vi "DAQmxAcqMessageLoop.vi"(8 "Error In":errorcluster, 11 "CommunicationRefs":T1) -> (0 "Error Out":errorcluster)   [LabVIEW 2015]
uses:
  TypeDefs/CommunicationRefs.ctl
  TypeDefs/MessageCluster.ctl
  TypeDefs/DAQmxAcqSettings.ctl
  <vilib>/DAQmx/read.llb/DAQmx Read (Analog 1D DBL 1Chan NSamp).vi
  <vilib>/Analysis/baseanly.llb/Mean (DBL).vi
  <vilib>/DAQmx/create/channels.llb/DAQmx Create Channel (AI-Temperature-Thermocouple).vi
  <vilib>/DAQmx/configure/timing.llb/DAQmx Timing (Sample Clock).vi
  <vilib>/DAQmx/miscellaneous.llb/DAQmx Fill In Error Info.vi
  <vilib>/Analysis/NI_AALBase.lvlib
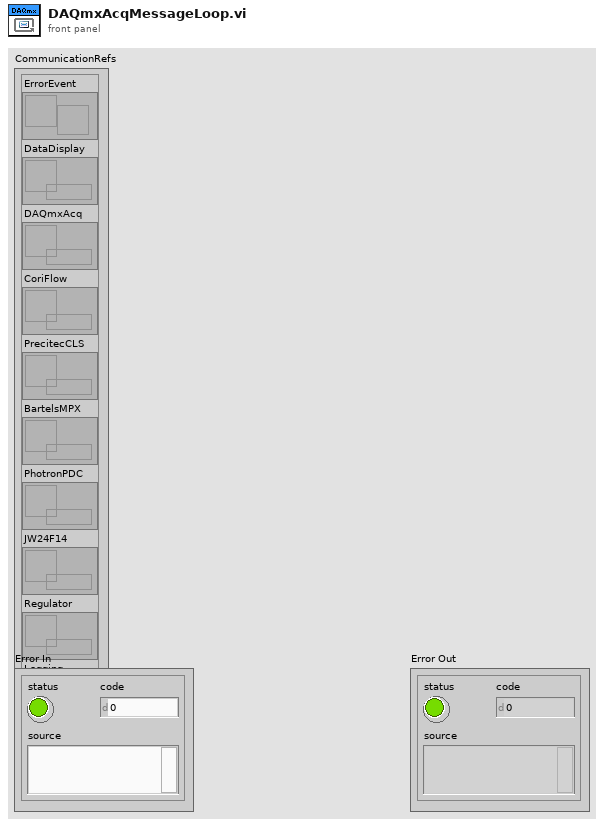
[diagram p1: front panel]
types:
  T1 = typedef "CommunicationRefs.ctl" = cluster{"ErrorEvent":refnum<user-event>, "DataDisplay":refnum<queue>, "DAQmxAcq":refnum<queue>, "CoriFlow":refnum<queue>, "PrecitecCLS":refnum<queue>, "BartelsMPX":refnum<queue>, "PhotronPDC":refnum<queue>, "JW24F14":refnum<queue>, "Regulator":refnum<queue>, "Logging":refnum<queue>}
  T2 = typedef "DAQmxAcqSettings.ctl" = cluster{"DAQmx Channel":tag, "Min Temp":dbl, "Max Temp":dbl, "Thermocouple Type":i32, "Simulate":bool, "Temp Unit":i32}
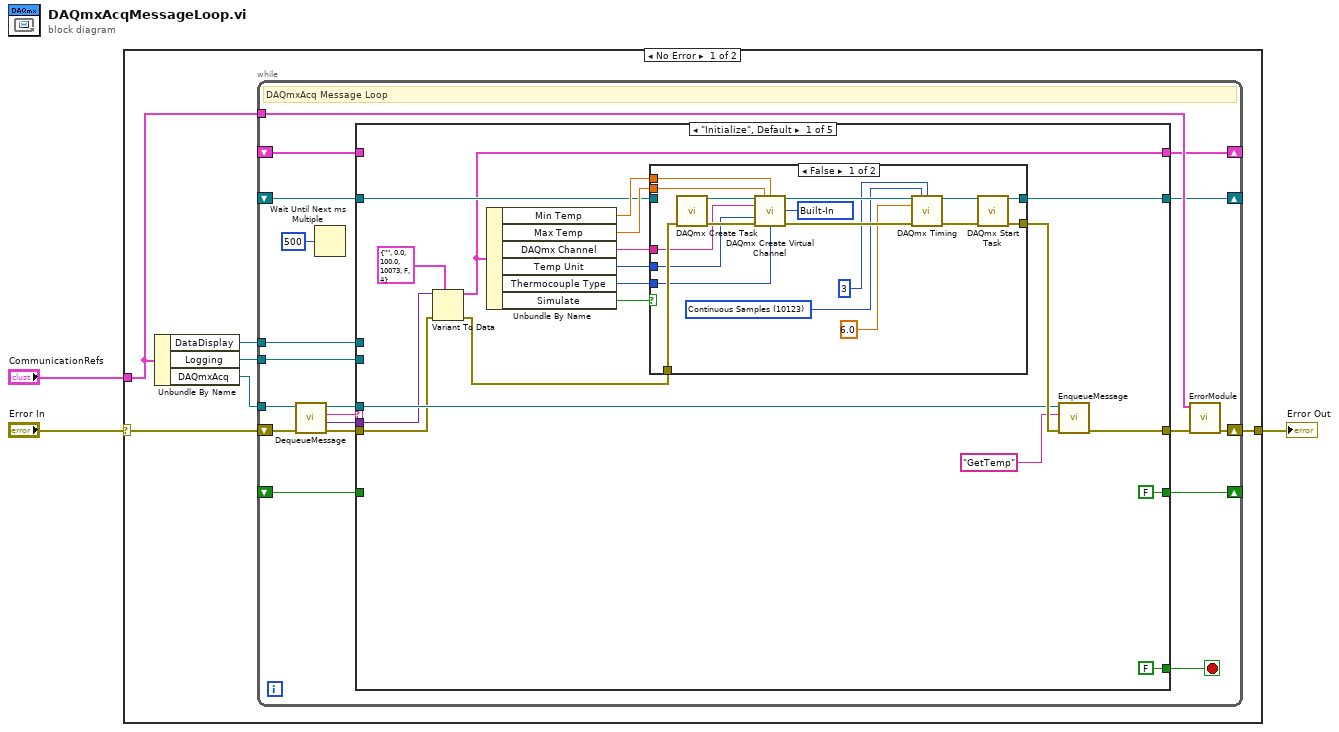
[diagram p0: block diagram]
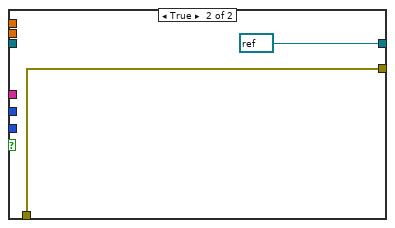
[diagram p2: hidden frame]
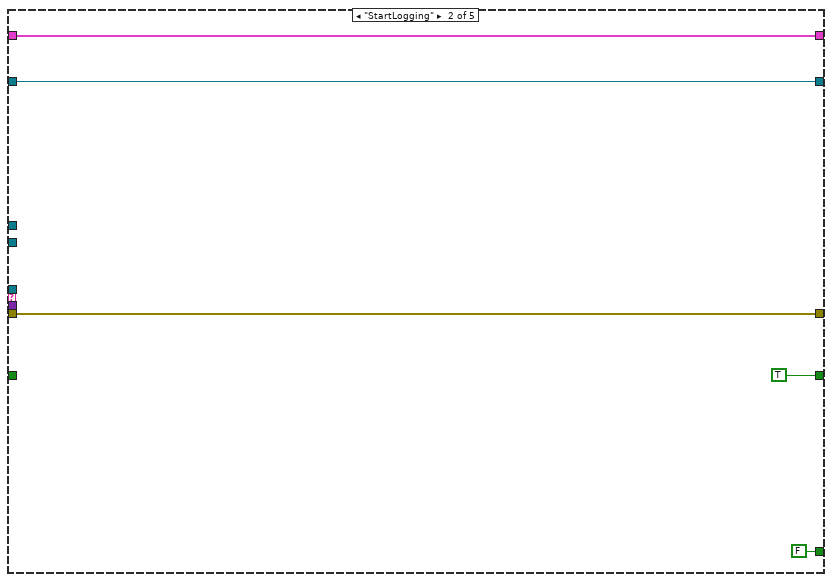
[diagram p3: hidden frame]
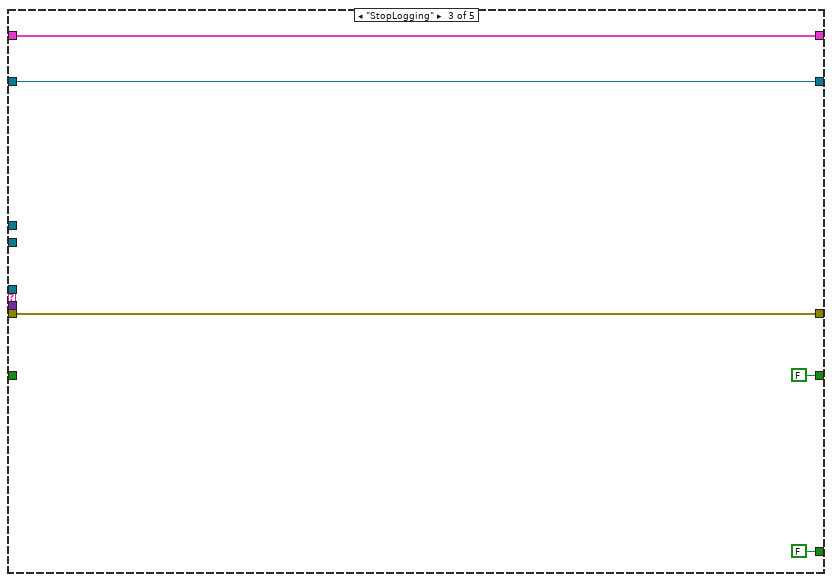
[diagram p4: hidden frame]
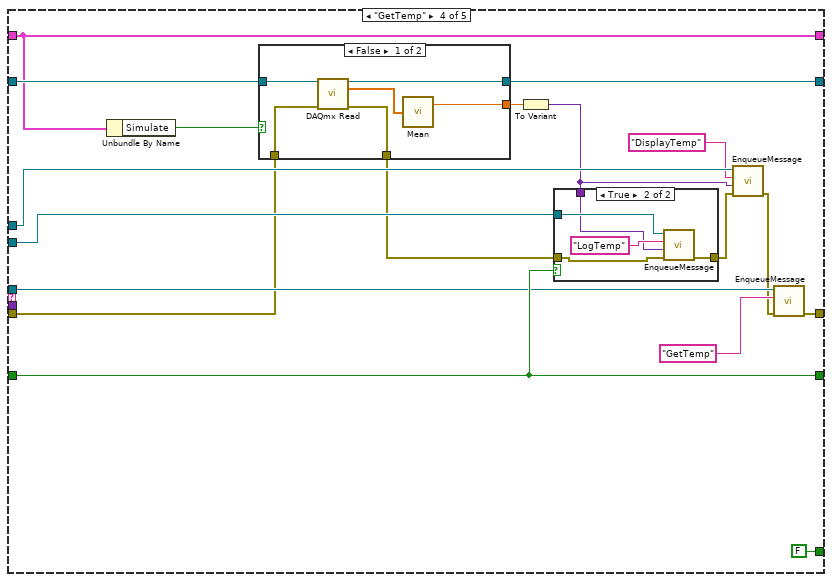
[diagram p5: hidden frame]
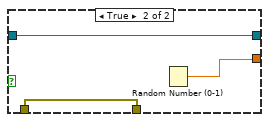
[diagram p6: hidden frame]
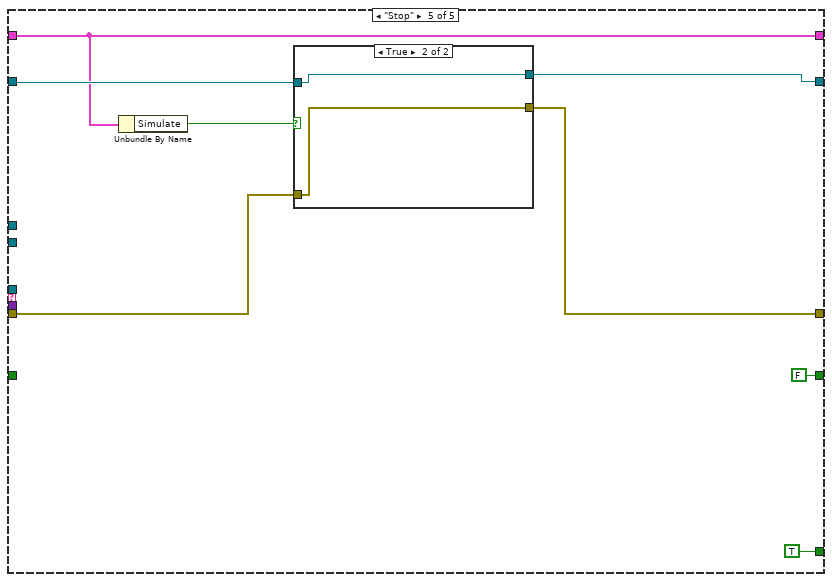
[diagram p8: hidden frame]
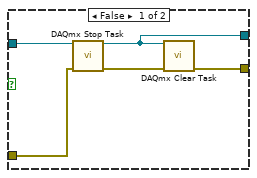
[diagram p9: hidden frame]
diagram:
  n1 = case shown="No Error" "Error In" {
    selector: "Error In" -> [w8 w126]
    tunnel: [w7 w126] -> w2
    tunnel: "CommunicationRefs" -> [w6 _]
    frame No Error {
      n2 = Unbundle By Name(w6) -> ("DataDisplay"=w5:refnum<queue>, "Logging"=w4:refnum<queue>, "DAQmxAcq"=w9:refnum<queue>)
      n3 = while {
        tunnel: w9 -> [w28]
        tunnel: w6 -> [w20]
        shift-right: [w22] -> w7
        shift-left: w8 -> [w27]
        tunnel: w5 -> [w18]
        tunnel: w4 -> [w17]
        shift-right: [w16] -> _
        shift-left: _ -> [w15]
        shift-right: [w14] -> _
        shift-left: _ -> [w13]
        shift-right: [w12] -> _
        shift-left: _ -> [w11]
        stop <- w19 stop-if-true
        # "DAQmxAcq Message Loop"
        n4 = call "DequeueMessage.vi"("error in (no error)"=w27, "MessageQueue"=w28) -> ("error out"=w23:errorcluster, "MessageData"=w24:variant, "Message"=w25:string, "dupMessageQueue"=w26:refnum<queue>)  [unwired: 6 in]
        n5 = Wait Until Next ms Multiple(millisecond multiple=u32 500) -> ()  [unwired: 1 out]
        n6 = case shown="\"Initialize\", Default" w25 {
          tunnel: w26 -> [w43 _ _ w87 _]
          tunnel: w24 -> [w40 _ _ _ _]
          tunnel: w23 -> [w41 w71 w77 w81 w112]
          tunnel: [w44 w71 w77 w88 w111] -> w21
          tunnel: [FALSE FALSE FALSE FALSE TRUE] -> w19
          tunnel: w18 -> [_ _ _ w94 _]
          tunnel: w17 -> [_ _ _ w95 _]
          tunnel: [FALSE TRUE FALSE w91 FALSE] -> w16
          tunnel: w15 -> [_ _ _ w91 _]
          tunnel: [w39 w69 w74 w82 w115] -> w14
          tunnel: w13 -> [w34 w69 w74 w90 w116]
          tunnel: [w32 w68 w73 w83 w114] -> w12
          tunnel: w11 -> [_ w68 w73 w83 w114]
          frame "Initialize", Default {
            n7 = Variant To Data(error in=w41, type=T2 {"DAQmx Channel"="", "Min Temp"=0.0, "Max Temp"=100.0, "Thermocouple Type"=10073, "Simulate"=FALSE, "Temp Unit"=4} ("DAQmxAcq Settings"), Variant=w40) -> (data=w32:T2, error out=w38:errorcluster)
            n8 = Unbundle By Name(w32) -> ("Min Temp"=w37:dbl, "Max Temp"=w36:dbl, "DAQmx Channel"=w35:tag, "Temp Unit"=w30:i32, "Thermocouple Type"=w31:i32, "Simulate"=w29:bool)
            n9 = case shown="False" w29 {
              tunnel: [w59 w67] -> w45
              tunnel: [w58 refnum<k21> refnum ("task out")] -> w39
              tunnel: w38 -> [w57 w67]
              tunnel: w37 -> [w56 _]
              tunnel: w36 -> [w55 _]
              tunnel: w35 -> [w54 _]
              tunnel: w34 -> [_ _]
              tunnel: w31 -> [w49 _]
              tunnel: w30 -> [w48 _]
              frame False {
                w51 = 10123 items=["Finite Samples"=10178, "Continuous Samples"=10123, "Hardware Timed Single Point"=12522] ("sample mode")
                w53 = 10200 items=["Built-In"=10200, "Constant Value"=10116, "Channel"=10113] ("cjc source")
                n10 = call <vilib>:"DAQmx Create Task.vi"("error in"=w57) -> ("task out"=w65:refnum<k21>, "error out"=w62:errorcluster)  [unwired: 13 in]
                n11 = call-poly <vilib>:"DAQmx Create Virtual Channel.vi"("task in"=w65, "maximum value"=w55, "minimum value"=w56, "physical channels"=w54, "cjc source"=w53, "units"=w48, "error in"=w62, "thermocouple type"=w49) -> ("task out"=w64:refnum<k21>, "error out"=w61:errorcluster)  [unwired: 6 in]
                n12 = call-poly <vilib>:"DAQmx Timing.vi"("task/channels in"=w64, "sample mode"=w51, "samples per channel"=3, "rate"=6.0, "error in"=w61) -> ("task out"=w63:refnum<k21>, "error out"=w60:errorcluster)  [unwired: 9 in]
                n13 = call <vilib>:"DAQmx Start Task.vi"("task/channels in"=w63, "error in"=w60) -> ("task out"=w58:refnum<k21>, "error out"=w59:errorcluster)  [unwired: 12 in]
              }
              frame True {
              }
            }
            n14 = call "EnqueueMessage.vi"("error in (no error)"=w45, "Message"="GetTemp", "MessageQueue"=w43) -> ("error out"=w44:errorcluster)  [unwired: 7 in, 1 out]
          }
          frame "StartLogging" {
          }
          frame "StopLogging" {
          }
          frame "GetTemp" {
            n15 = Unbundle By Name(w83) -> ("Simulate"=w89:bool)
            n16 = case shown="False" w89 {
              tunnel: w90 -> [w100 w103]
              tunnel: [w99 w104] -> w85
              tunnel: [w98 w103] -> w82
              tunnel: w81 -> [w97 w102]
              tunnel: [w96 w102] -> w80
              frame False {
                n17 = call-poly <vilib>:"DAQmx Read.vi"("task/channels in"=w100, "error in"=w97) -> ("task out"=w98:refnum<k21>, "data"=w101:dbl[], "error out"=w96:errorcluster)  [unwired: 11 in]
                n18 = call-poly <vilib>:"Mean.vi"("X"=w101) -> ("mean"=w99:dbl)  [unwired: 1 out]
              }
              frame True {
                n19 = Random Number (0-1)() -> (number: 0 to 1=w104:dbl)
              }
            }
            n20 = To Variant(anything=w85) -> (Variant=w84:variant)
            n21 = case shown="True" w91 {
              tunnel: w95 -> [_ w110]
              tunnel: w80 -> [w105 w107]
              tunnel: [w105 w106] -> w79
              tunnel: w84 -> [_ w108]
              frame False {
              }
              frame True {
                n22 = call "EnqueueMessage.vi"("error in (no error)"=w107, "MessageData"=w108, "Message"="LogTemp", "MessageQueue"=w110) -> ("error out"=w106:errorcluster)  [unwired: 6 in, 1 out]
              }
            }
            n23 = call "EnqueueMessage.vi"("error in (no error)"=w79, "MessageData"=w84, "Message"="DisplayTemp", "MessageQueue"=w94) -> ("error out"=w78:errorcluster)  [unwired: 6 in, 1 out]
            n24 = call "EnqueueMessage.vi"("error in (no error)"=w78, "Message"="GetTemp", "MessageQueue"=w87) -> ("error out"=w88:errorcluster)  [unwired: 7 in, 1 out]
          }
          frame "Stop" {
            n25 = Unbundle By Name(w114) -> ("Simulate"=w113:bool)
            n26 = case shown="True" w113 {
              tunnel: w116 -> [w123 w124]
              tunnel: [w122 w124] -> w115
              tunnel: w112 -> [w121 w125]
              tunnel: [w119 w125] -> w111
              frame False {
                n27 = call <vilib>:"DAQmx Stop Task.vi"("task/channels in"=w123, "error in"=w121) -> ("task out"=w122:refnum<k21>, "error out"=w120:errorcluster)  [unwired: 12 in]
                n28 = call <vilib>:"DAQmx Clear Task.vi"("task in"=w122, "error in"=w120) -> ("error out"=w119:errorcluster)  [unwired: 13 in]
              }
              frame True {
              }
            }
          }
        }
        n29 = call "ErrorModule.vi"("Error In"=w21, "CommunicationRefs"=w20) -> ("Error Out"=w22:errorcluster)  [unwired: 9 in]
      }
    }
    frame Error {
    }
  }
  "Error Out" <- w2
